vi "Cam.vi"() -> ()   [LabVIEW 2021]
uses:
  <vilib>/userdefined/High Color/IMAQdx.ctl
  <vilib>/vision/driver/NI_Vision_Acquisition_Software.lvlib
  <vilib>/vision/NI_Vision_Development_Module.lvlib
panel:
  out "EJE Y":sgl
  out "EJE X":sgl
  in  "Reconocer":bool
  out "Muestra":T1(plugin-control)
  out "Imagen":T1(plugin-control)
  in  "Camara":T2
  in  "stop":bool
  # "ELECTROMARK VISION ARTIFICIAL"
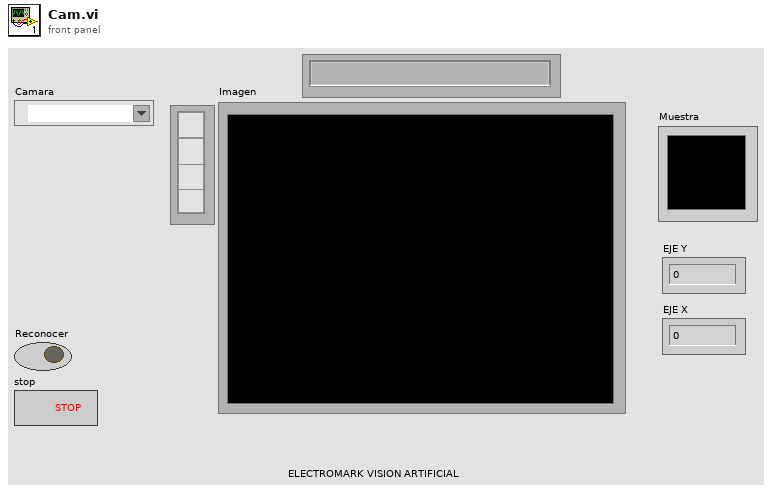
[diagram p1: front panel]
types:
  T1 = typedef "IMAQ Image.ctl" = refnum<image>
  T2 = typedef "IMAQdx.ctl" = refnum<k21>
  T3 = typedef "Image Type" = u32
  T4 = cluster{"Match Mode":u16, "Number of Matches Requested":i32, "Minimum Match Score":sgl, "SubPixel Accuracy":bool, "Rotation Angle Ranges":cluster{"Start":sgl, "End":sgl}[], "Show Search Area":bool, "Show Result":bool}
  T5 = cluster{"Position":cluster{"x":sgl, "y":sgl}, "Angle":sgl, "Scale":sgl, "Score":sgl, "Bounding Box":cluster{"x":sgl, "y":sgl}[]}[]
  T6 = cluster{"Matches[0]":cluster{"Position":cluster{"x":sgl, "y":sgl}, "Angle":sgl, "Scale":sgl, "Score":sgl, "Bounding Box":cluster{"x":sgl, "y":sgl}[]}, "Matches[1]":cluster{"Position":cluster{"x":sgl, "y":sgl}, "Angle":sgl, "Scale":sgl, "Score":sgl, "Bounding Box":cluster{"x":sgl, "y":sgl}[]}, "Matches[2]":cluster{"Position":cluster{"x":sgl, "y":sgl}, "Angle":sgl, "Scale":sgl, "Score":sgl, "Bounding Box":cluster{"x":sgl, "y":sgl}[]}, "Matches[3]":cluster{"Position":cluster{"x":sgl, "y":sgl}, "Angle":sgl, "Scale":sgl, "Score":sgl, "Bounding Box":cluster{"x":sgl, "y":sgl}[]}, "Matches[4]":cluster{"Position":cluster{"x":sgl, "y":sgl}, "Angle":sgl, "Scale":sgl, "Score":sgl, "Bounding Box":cluster{"x":sgl, "y":sgl}[]}, "Matches[5]":cluster{"Position":cluster{"x":sgl, "y":sgl}, "Angle":sgl, "Scale":sgl, "Score":sgl, "Bounding Box":cluster{"x":sgl, "y":sgl}[]}, "Matches[6]":cluster{"Position":cluster{"x":sgl, "y":sgl}, "Angle":sgl, "Scale":sgl, "Score":sgl, "Bounding Box":cluster{"x":sgl, "y":sgl}[]}, "Matches[7]":cluster{"Position":cluster{"x":sgl, "y":sgl}, "Angle":sgl, "Scale":sgl, "Score":sgl, "Bounding Box":cluster{"x":sgl, "y":sgl}[]}, "Matches[8]":cluster{"Position":cluster{"x":sgl, "y":sgl}, "Angle":sgl, "Scale":sgl, "Score":sgl, "Bounding Box":cluster{"x":sgl, "y":sgl}[]}}
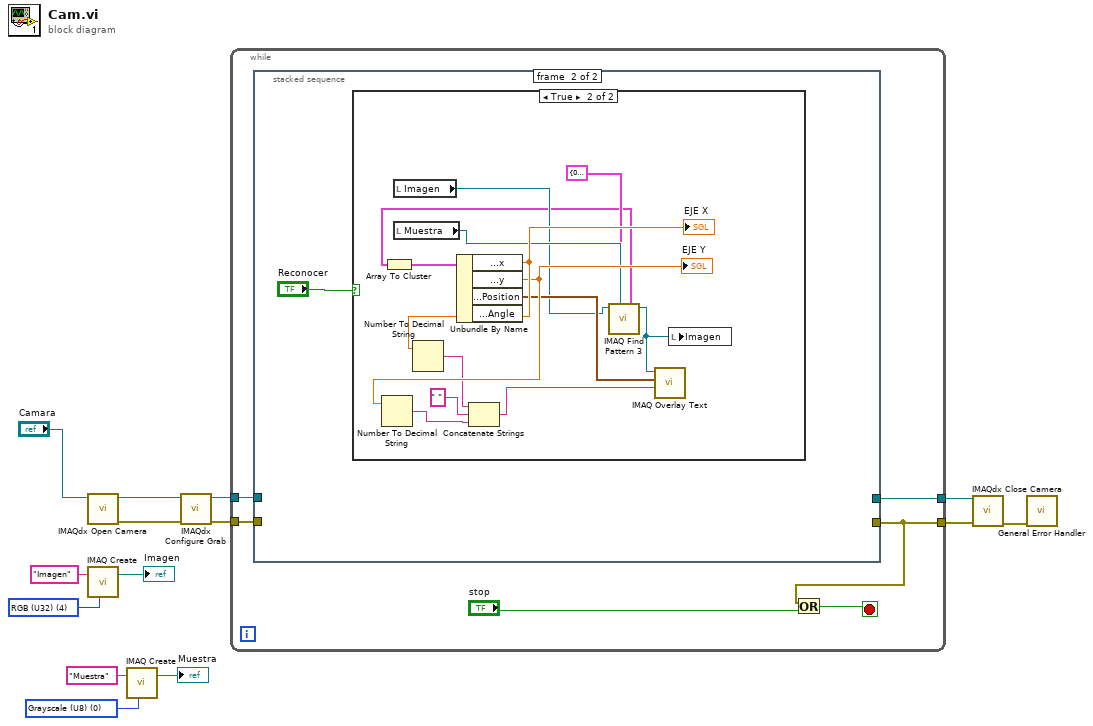
[diagram p0: block diagram]
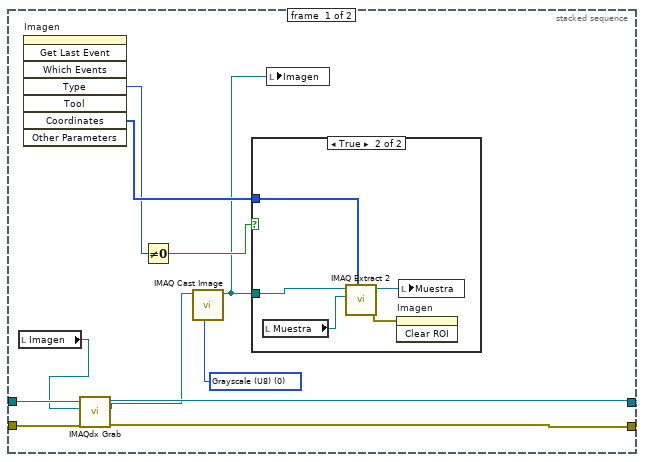
[diagram p2: hidden frame]
diagram:
  w5 = T3 0 items=["Grayscale (U8)", "Grayscale (I16)", "Grayscale (SGL)", "Complex (CSG)", "RGB (U32)", "HSL (U32)", "RGB (U64)", "Grayscale (U16)"] ("Image Type")
  w8 = T3 4 items=["Grayscale (U8)", "Grayscale (I16)", "Grayscale (SGL)", "Complex (CSG)", "RGB (U32)", "HSL (U32)", "RGB (U64)", "Grayscale (U16)"] ("Image Type")
  n1 = call <vilib>:"IMAQdx Open Camera.vi"("Session In"="Camara") -> ("error out"=w12:errorcluster, "Session Out"=w13:T2)  [unwired: 9 in]
  n2 = call "IMAQ Create"("Image Name"="Imagen", "Image Type"=w8) -> ("New Image"=→"Imagen":T1)  [unwired: 3 in, 1 out]
  n3 = call "IMAQ Create"("Image Name"="Muestra", "Image Type"=w5) -> ("New Image"=→"Muestra":T1)  [unwired: 3 in, 1 out]
  n4 = call <vilib>:"IMAQdx Configure Grab.vi"("error in"=w12, "Session In"=w13) -> ("error out"=w11:errorcluster, "Session Out"=w10:T2)  [unwired: 8 in]
  n5 = while {
    tunnel: w11 -> [w20]
    tunnel: w10 -> [w19]
    tunnel: [w18] -> w4
    tunnel: [w15] -> w3
    stop <- w17 stop-if-true
    n6 = stacked-sequence {
      tunnel: w20 -> [w31 _]
      tunnel: w19 -> [w30 _]
      tunnel: [w29 _] -> w18
      tunnel: [w28 _] -> w15
      frame #0 {
        w27 = T3 0 items=["Grayscale (U8)", "Grayscale (I16)", "Grayscale (SGL)", "Complex (CSG)", "RGB (U32)", "HSL (U32)", "RGB (U64)", "Grayscale (U16)"] ("Image Type")
        n7 = local read "Imagen"() -> (w24:T1)
        n8 = invoke on="Imagen" class="ImageControl" method="Get Last Event"() -> ("Type"=w22:i32, "Coordinates"=w26:i32[])  [unwired: 8 in, 6 out]
        n9 = call <vilib>:"IMAQdx Grab.vi"("error in"=w31, "Image In"=w24, "Session In"=w30) -> ("error out"=w28:errorcluster, "Image Out"=w21:T1, "Session Out"=w29:T2)  [unwired: 5 in, 1 out]
        n10 = Not Equal To 0?(x=w22) -> (x != 0?=w25:bool)
        n11 = call "IMAQ Cast Image"("Image Type"=w27, "Image Src"=w21) -> ("Image Dst Out"=w23:T1)  [unwired: 8 in, 1 out]
        n12 = case shown="True" w25 {
          tunnel: w23 -> [_ w35]
          tunnel: w26 -> [_ w36]
          frame False {
          }
          frame True {
            n13 = local read "Muestra"() -> (w33:T1)
            n14 = call "IMAQ Extract 2"("Optional Rectangle"=w36, "Image Dst"=w33, "Image Src"=w35) -> ("error out"=w32:errorcluster, "Image Dst Out"=w34:T1)  [unwired: 7 in]
            n15 = invoke on="Imagen" class="ImageControl" method="Clear ROI"(error in=w32) -> ()  [unwired: 2 in, 3 out]
            n16 = local write "Muestra"(w34) -> ()
          }
        }
        n17 = local write "Imagen"(w23) -> ()
      }
      frame #1 {
        n18 = case shown="True" "Reconocer" {
          frame False {
          }
          frame True {
            n19 = local read "Imagen"() -> (w41:T1)
            n20 = local read "Muestra"() -> (w42:T1)
            n21 = call "IMAQ Find Pattern 3"("Settings"=T4 {"Match Mode"=0, "Number of Matches Requested"=1, "Minimum Match Score"=800.0, "SubPixel Accuracy"=FALSE, "Rotation Angle Ranges"=[], "Show Search Area"=TRUE, "Show Result"=TRUE}, "Template"=w42, "Image"=w41) -> ("Image Out"=w39:T1, "Matches"=w38:T5)  [unwired: 3 in, 4 out]
            n22 = Array To Cluster(array=w38) -> (cluster=w50:T6)
            n23 = Unbundle By Name(w50) -> ("Matches[0].Position.x"=w49:sgl, "Matches[0].Position.y"=w48:sgl, "Matches[1].Position"=w46:cluster{"x":sgl, "y":sgl})  [unwired: 1 out]
            "EJE X" <- w49
            "EJE Y" <- w48
            n24 = Number To Decimal String(number=w48) -> (decimal integer string=w44:string)  [unwired: 1 in]
            n25 = Number To Decimal String(number=w49) -> (decimal integer string=w47:string)  [unwired: 1 in]
            n26 = Concatenate Strings(w47, " " ("string"), w44) -> (w45:string)
            n27 = call "IMAQ Overlay Text"("String"=w45, "Origin"=w46, "Image"=w39) -> ()  [unwired: 7 in, 2 out]
            n28 = local write "Imagen"(w39) -> ()
          }
        }
      }
    }
    n29 = Or(x=w15, y="stop") -> (x .or. y?=w17:bool)
  }
  n30 = call <vilib>:"IMAQdx Close Camera.vi"("error in"=w3, "Session In"=w4) -> ("error out"=w7:errorcluster)  [unwired: 9 in]
  n31 = call <vilib>:"General Error Handler.vi"("error in (no error)"=w7) -> ()  [unwired: 10 in, 5 out]
